vi "WiFi HttpsUpload_CameraPhoto2Telegram.vi"   [LabVIEW 2014]
uses:
  <vilib>/Aledyne-TSXperts/Arduino Compatible Compiler for LabVIEW/Code Generator/Arduino APIs/Digital/PinDirection.ctl
  QwaveSys_ESP8266/QwaveSys_ESP8266.lvlib
  QwaveSys_Interface/QwaveSys_Interface.lvlib
  <vilib>/Aledyne-TSXperts/Arduino Compatible Compiler for LabVIEW/Arduino Compatible Compiler for LabVIEW.lvlib
types:
  T1 = typedef "Arduino Compatible Compiler for LabVIEW.lvlib/PinDirection.ctl" = enum16{" INPUT", "OUTPUT", " INPUT_PULLUP"}
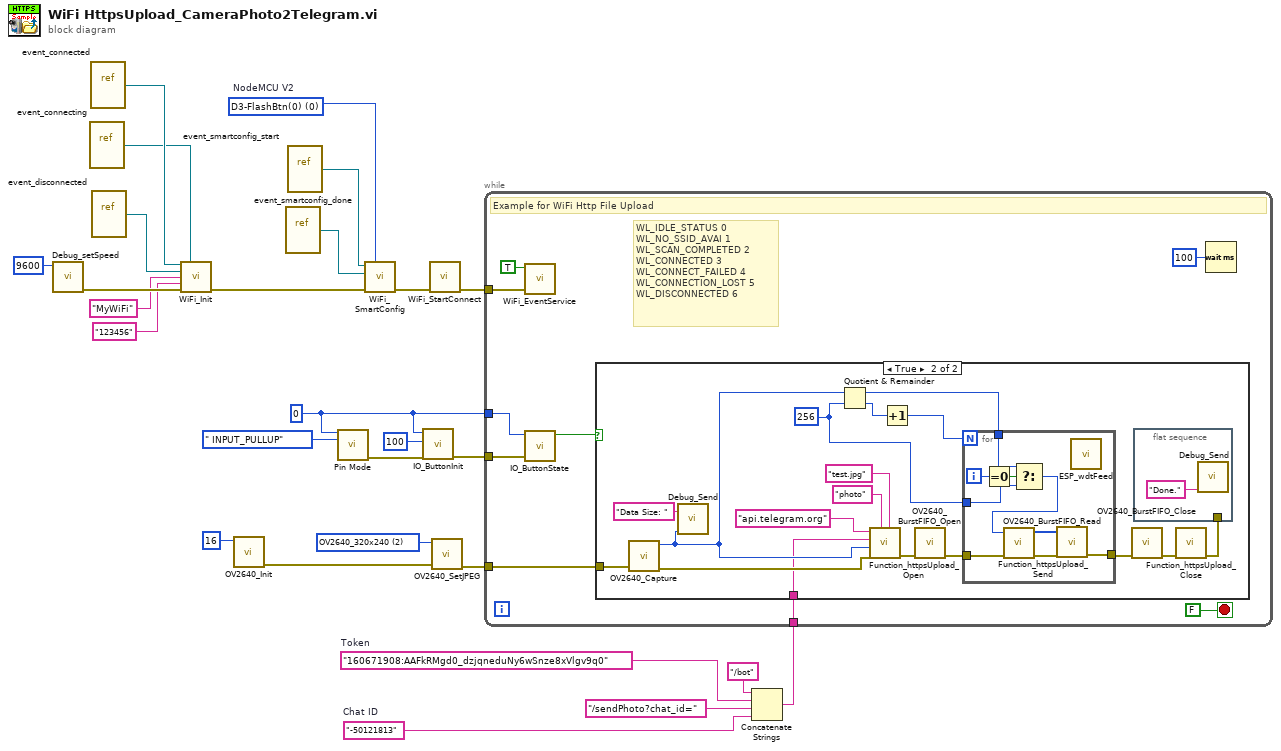
[diagram p0: block diagram]
diagram:
  w2 = "160671908:AAFkRMgd0_dzjqneduNy6wSnze8xVlgv9q0"  # Token
  w1 = "-50121813"  # Chat ID
  w8 = u8 0 ("PIN")
  w13 = u16 2 items=["OV2640_160x120", "OV2640_176x144", "OV2640_320x240", "OV2640_352x288", "OV2640_640x480", "OV2640_800x600", "OV2640_1024x768", "OV2640_1280x1024", "OV2640_1600x1200"] ("resolution")
  w20 = u8 0 items=["D0-(LED)-(16)"=16, "D1-SCL(5)"=5, "D2-SDA(4)"=4, "D3-FlashBtn(0)"=0, "D4-(2)"=2, "D5-SCK(14)"=14, "D6-MISO(12)"=12, "D7-MOSI(13)"=13, "D8-SS(15)"=15, "D9-TX(3)"=3, "D10-RX(1)"=1, "ADC0,(17)"=17]  # NodeMCU V2
  n1 = call "Debug_setSpeed.vi"("Speed"=u32 9600) -> ("error out"=w22:errorcluster)  [unwired: 10 in]
  n2 = vi-ref "event_connecting.vi"() -> (w17:refnum<vi>)
  n3 = vi-ref "event_connected.vi"() -> (w18:refnum<vi>)
  n4 = vi-ref "event_disconnected.vi"() -> (w16:refnum<vi>)
  n5 = call "WiFi_Init.vi"("connected"=w18, "connecting"=w17, "disconnected"=w16, "SSID"="MyWiFi", "PASSPHARSE"="123456", "error in (no error)"=w22) -> ("error out"=w27:errorcluster)  [unwired: 9 in]
  n6 = call "OV2640_Init.vi"("CS"=u8 16) -> ("error out"=w12:errorcluster)  [unwired: 9 in, 1 out]
  n7 = vi-ref "event_smartconfig_done.vi"() -> (w23:refnum<vi>)
  n8 = vi-ref "event_smartconfig_start.vi"() -> (w24:refnum<vi>)
  n9 = call <vilib>:"Pin Mode.vi"("pin"=w8, "direction"=PinDirection." INPUT_PULLUP") -> ("error out"=w7:errorcluster)  [unwired: 13 in]
  n10 = call "WiFi_SmartConfig.vi"("Smart Config Enter Pin"=w20, "error in (no error)"=w27, "smartconfig_done"=w23, "smartconfig_start"=w24) -> ("error out"=w26:errorcluster)  [unwired: 7 in]
  n11 = call "IO_ButtonInit.vi"("error in (no error)"=w7, "debounce (ms)"=u16 100, "PIN"=w8) -> ("error out"=w9:errorcluster)  [unwired: 8 in]
  n12 = call "WiFi_StartConnect.vi"("error in (no error)"=w26) -> ("error out"=w25:errorcluster)  [unwired: 10 in]
  n13 = call "OV2640_SetJPEG.vi"("error in (no error)"=w12, "resolution"=w13) -> ("error out"=w11:errorcluster)  [unwired: 9 in]
  n14 = Concatenate Strings("/bot", w2, "/sendPhoto?chat_id=", w1) -> (w5:string)
  n15 = while {
    tunnel: w25 -> [w35]
    tunnel: w11 -> [w32]
    tunnel: w5 -> [w31]
    tunnel: w9 -> [w30]
    tunnel: w8 -> [w29]
    stop <- FALSE stop-if-true
    # "WL_IDLE_STATUS\t0\nWL_NO_SSID_AVAI\t1\nWL_SCAN_COMPLETED\t2\nWL_CONNECTED\t3\nWL_CONNECT_FAILED\t4\nWL_CONNECTION_LOST\t5\nWL_DISCONNECTED\t6"
    # "Example for WiFi Http File Upload"
    n16 = call "WiFi_EventService.vi"("error in (no error)"=w35, "wait for connected (True)"=TRUE) -> ()  [unwired: 8 in, 2 out]
    n17 = call "IO_ButtonState.vi"("error in (no error)"=w30, "PIN"=w29) -> ("State"=w28:bool)  [unwired: 8 in, 1 out]
    n18 = case shown="True" w28 {
      tunnel: w32 -> [_ w53]
      tunnel: w31 -> [_ w40]
      frame False {
      }
      frame True {
        w48 = u32 256 ("y")
        n19 = call "OV2640_Capture.vi"("error in (no error)"=w53) -> ("error out"=w41:errorcluster, "FIFO Length"=w42:u32)  [unwired: 9 in]
        n20 = call "Debug_Send.vi"("Name"="Data Size: ", "DATA"=w42) -> ()  [unwired: 10 in]
        n21 = Quotient & Remainder(x=w42, y=w48) -> (x-y*floor(x/y)=w49:u32, floor(x/y)=w52:u32)
        n22 = call "Function_httpsUpload_Open.vi"("Filename"="test.jpg", "Name"="photo", "error in (no error)"=w41, "Upload Lenght"=w42, "URI"=w40, "Host"="api.telegram.org") -> ("error out"=w46:errorcluster)  [unwired: 5 in]
        n23 = Increment(x=w52) -> (x+1=w50:u32)
        n24 = call "OV2640_BurstFIFO_Open.vi"("error in (no error)"=w46) -> ("error out"=w51:errorcluster)  [unwired: 10 in]
        n25 = for {
          N: w50 -> [_]
          tunnel: w51 -> [w63]
          tunnel: w49 -> [w60]
          tunnel: w48 -> [w59]
          tunnel: [w56] -> w39
          i -> [w62]
          n26 = Equal To 0?(x=w62) -> (x = 0?=w61:bool)
          n27 = Select(t=w60, s=w61, f=w59) -> (s? t:f=w55:u32)
          n28 = call "OV2640_BurstFIFO_Read.vi"("error in (no error)"=w63, "Lenght"=w55) -> ("error out"=w58:errorcluster, "DATA"=w57:u8[])  [unwired: 8 in]
          n29 = call "Function_httpsUpload_Send.vi"("error in (no error)"=w58, "DATA"=w57) -> ("error out"=w56:errorcluster)  [unwired: 9 in]
          n30 = call "ESP_wdtFeed.vi"() -> ()  [unwired: 11 in, 1 out]
        }
        n31 = call "OV2640_BurstFIFO_Close.vi"("error in (no error)"=w39) -> ("error out"=w38:errorcluster)  [unwired: 10 in]
        n32 = flat-sequence {
          tunnel: w37 -> [_]
          frame #0 {
            n33 = call "Debug_Send.vi"("DATA"="Done." ("Name")) -> ()  [unwired: 11 in]
          }
        }
        n34 = call "Function_httpsUpload_Close.vi"("error in (no error)"=w38) -> ("error out"=w37:errorcluster)  [unwired: 10 in]
      }
    }
    n35 = Wait (ms)(milliseconds to wait=u32 100) -> ()  [unwired: 1 out]
  }
